vi "Configure Digital Gen Sine.vi"(0 "VISA resource name":refnum<visa-resource-name>, 1 "Frequency (10 Hz)":dbl=10.0, 2 "Enable Waveform (T: Enable)":bool=TRUE, 5 "Channel (0: chA)":i32(ring) items=["chA", "chB"], 7 "Type (0: Sine)":i32(ring) items=["Sine", "PhasedSine"], 9 "Amplitude (0 FFS)":dbl, 11 "error in (no error)":errorcluster, 12 "Enable EQ Output Modification (T: Enable)":bool=TRUE, 13 "Phase Difference (0 degrees)":dbl) -> (4 "VISA resource name out":refnum<visa-resource-name>, 15 "error out":errorcluster)   [LabVIEW 2014, in "Stanford Research SR1.lvlib"]
doc: "Configures the attributes for the Digital Generator Sine."
uses:
  Stanford Research SR1.lvlib
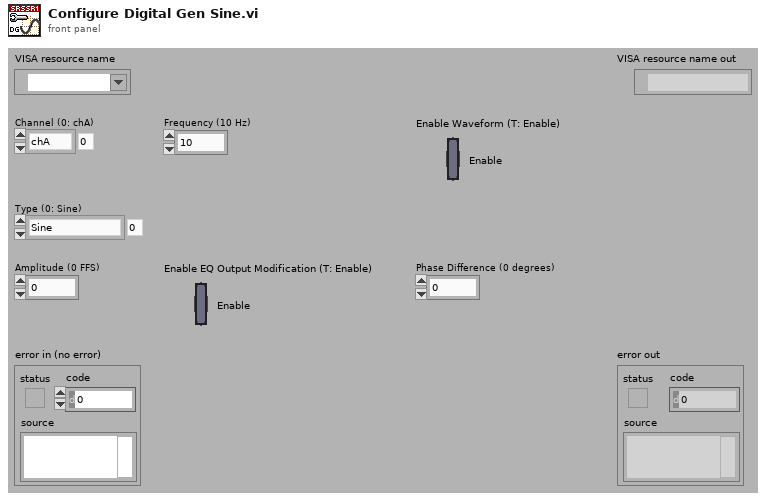
[diagram p1: front panel]
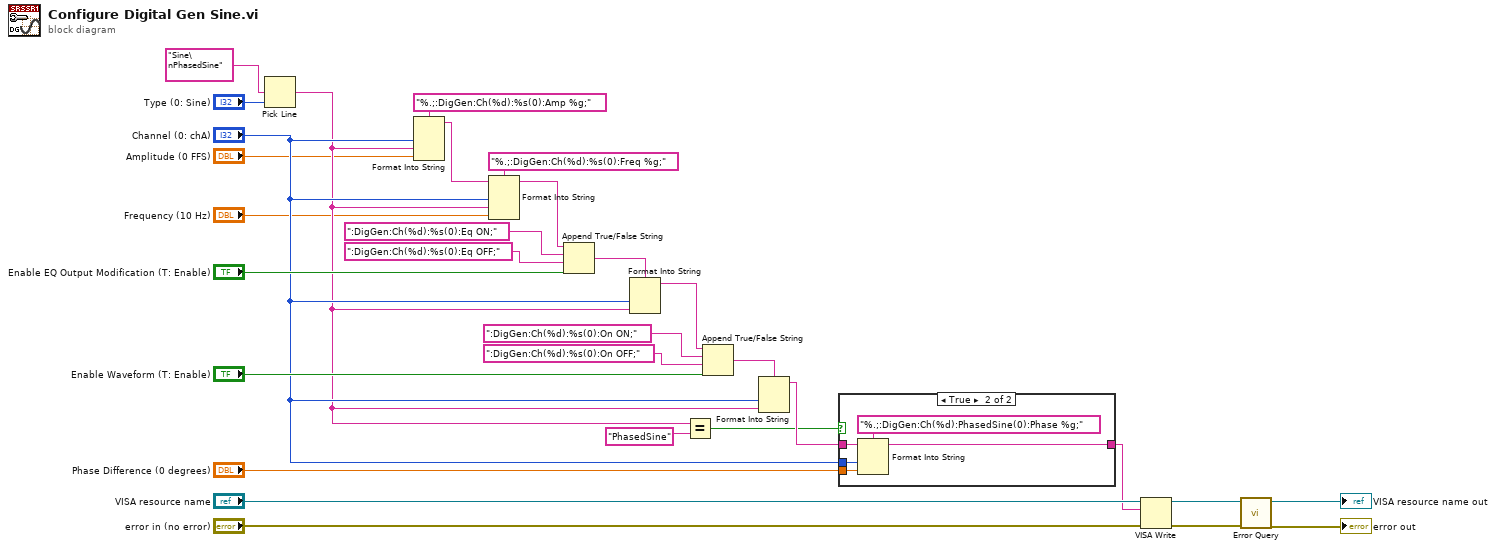
[diagram p0: block diagram]
diagram:
  n1 = Pick Line(multi-line string="Sine\nPhasedSine" ("string (\"\")"), line index="Type (0: Sine)") -> (output string=w4:string)  [unwired: 1 in]
  n2 = Format Into String(format string="%.;:DigGen:Ch(%d):%s(0):Amp %g;", "Channel (0: chA)", w4, "Amplitude (0 FFS)") -> (resulting string=w29:string)  [unwired: 2 in, 1 out]
  n3 = Format Into String(format string="%.;:DigGen:Ch(%d):%s(0):Freq %g;", initial string=w29, "Channel (0: chA)", w4, "Frequency (10 Hz)") -> (resulting string=w27:string)  [unwired: 1 in, 1 out]
  n4 = Append True/False String(1:"Enable EQ Output Modification (T: Enable)", 2:":DigGen:Ch(%d):%s(0):Eq OFF;", 3:":DigGen:Ch(%d):%s(0):Eq ON;", 4:w27) -> (0:w14:string)
  n5 = Format Into String(format string=w14, "Channel (0: chA)", w4) -> (resulting string=w13:string)  [unwired: 2 in, 1 out]
  n6 = Equal?(x=w4, y="PhasedSine") -> (x = y?=w6:bool)
  n7 = Append True/False String(1:"Enable Waveform (T: Enable)", 2:":DigGen:Ch(%d):%s(0):On OFF;", 3:":DigGen:Ch(%d):%s(0):On ON;", 4:w13) -> (0:w12:string)
  n8 = Format Into String(format string=w12, "Channel (0: chA)", w4) -> (resulting string=w11:string)  [unwired: 2 in, 1 out]
  n9 = case shown="True" w6 {
    tunnel: w11 -> [w31 w35]
    tunnel: "Channel (0: chA)" -> [_ w34]
    tunnel: [w31 w33] -> w9
    tunnel: "Phase Difference (0 degrees)" -> [_ w32]
    frame False {
    }
    frame True {
      n10 = Format Into String(format string="%.;:DigGen:Ch(%d):PhasedSine(0):Phase %g;", initial string=w35, w34, w32) -> (resulting string=w33:string)  [unwired: 1 in, 1 out]
    }
  }
  n11 = VISA Write(VISA resource name="VISA resource name", write buffer=w9, error in (no error)="error in (no error)") -> (VISA resource name out=w18:refnum<visa-resource-name>, error out=w17:errorcluster)  [unwired: 1 out]
  n12 = call "Error Query.vi"("error in (no error)"=w17, "VISA resource name"=w18) -> ("error out"=→"error out":errorcluster, "VISA resource name out"=→"VISA resource name out":refnum<visa-resource-name>)  [unwired: 6 in, 2 out]
